vi "Read File Contents.vi"(8 "error in (no error)":errorcluster, 11 "File Name":string) -> (0 "error out":errorcluster, 3 "File Text":string)   [LabVIEW 2017, in "TestTextFileSink.lvclass"]
uses:
  TestTextFileSink.lvclass
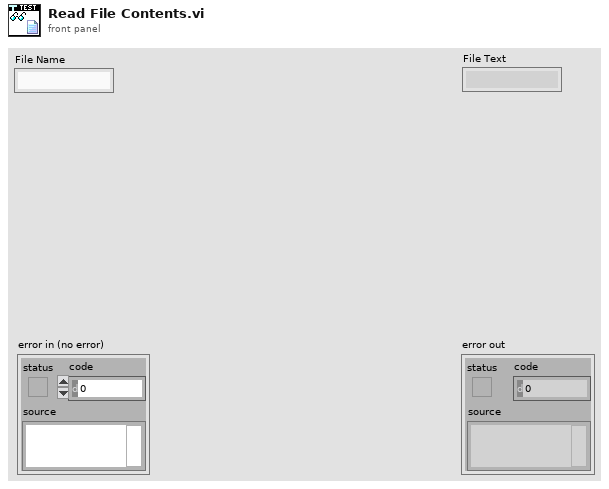
[diagram p1: front panel]
types:
  T1 = enum16{"open", "replace", "create", "open or create", "replace or create", "replace or create with confirmation"}
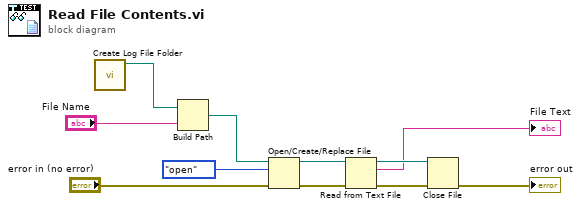
[diagram p0: block diagram]
diagram:
  n1 = call "Create Log File Folder.vi"() -> ("Folder Path"=w11:path)  [unwired: 10 in, 1 out]
  n2 = Build Path(base path=w11, name or relative path="File Name") -> (appended path=w9:path)
  n3 = Open/Create/Replace File(file path (use dialog)=w9, error in="error in (no error)", operation (0:open)=T1."open") -> (refnum out=w6:refnum<file>, error out=w5:errorcluster)  [unwired: 3 in, 1 out]
  n4 = Read from Text File(file (use dialog)=w6, error in=w5) -> (refnum out=w4:refnum<file>, text=→"File Text":string, error out=w3:errorcluster)  [unwired: 2 in, 1 out]
  n5 = Close File(refnum=w4, error in=w3) -> (error out=→"error out":errorcluster)  [unwired: 1 out]
